vi "User Event IO.vi"() -> ()   [LabVIEW 2017]
uses:
  IMAQCV/GPIO/GPIO Pins.ctl
  <vilib>/Platform/TimedLoop/XDataNode/timing_clust.ctl
  <vilib>/Platform/TimedLoop/XDataNode/nitl_modes.ctl
  <vilib>/Platform/TimedLoop/XDataNode/wakeup.ctl
  <vilib>/platform/TimedLoop/XDataNode/XDataNode.xnode
  <vilib>/Platform/TimedLoop/XDataNode/XDNodeRunTimeDep.lvlib
  IMAQCV/PIIO.lvlib
panel:
  out "DIO4":bool
  out "DIO3":bool
  out "DIO2":bool
  out "DIO1":bool
  in  "stop":bool
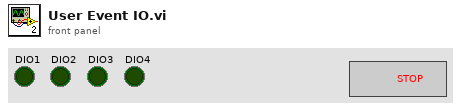
[diagram p1: front panel]
types:
  T1 = typedef "PIIO.lvlib/GPIO Pins.ctl" = u8
  T2 = cluster{"GPIO":T1[], "MODE":enum8{"INPUT", "OUTPUT"}[]}
  T3 = typedef "XDNodeRunTimeDep.lvlib/timing_clust.ctl" = cluster{"Expected End [f-1]":u64, "Actual End [f-1]":u64, "Finished Late? [f-1]":bool, "Expected End [i-1]":u64, "Actual End [i-1]":u64, "Finished Late? [i-1]":bool, "Expected Start [i]":u64, "Actual Start [i]":u64, "Expected Start [f]":u64, "Actual Start [f]":u64, "Source Name":string, "Structure Name":string, "Period":i64, "Deadline":i64, "Offset":i64, "Start":i64, "Priority":i32, "Timeout":i32, "Mode":T4, "Wakeup Reason":T5, "Error":errorcluster, "Source Type":string, "Secondary Source Type":string, "Global End Time":u64, "Global Start Time":u64, "Frame Duration":u64, "Iteration Duration":u64, "Assigned CPU":i32, "I/O Scan Engine Mode":u32}
  T4 = typedef "XDNodeRunTimeDep.lvlib/nitl_modes.ctl" = enum32{"No Change", "Process missed periods, maintain original phase", "Discard missed periods, maintain original phase", "Process missed periods, ignore original phase", "Discard missed periods, ignore original phase"}
  T5 = typedef "XDNodeRunTimeDep.lvlib/wakeup.ctl" = enum32{"Normal", "Aborted", "Asynchronous wakeup", "Timing source error", "Timed loop error", "Timeout"}
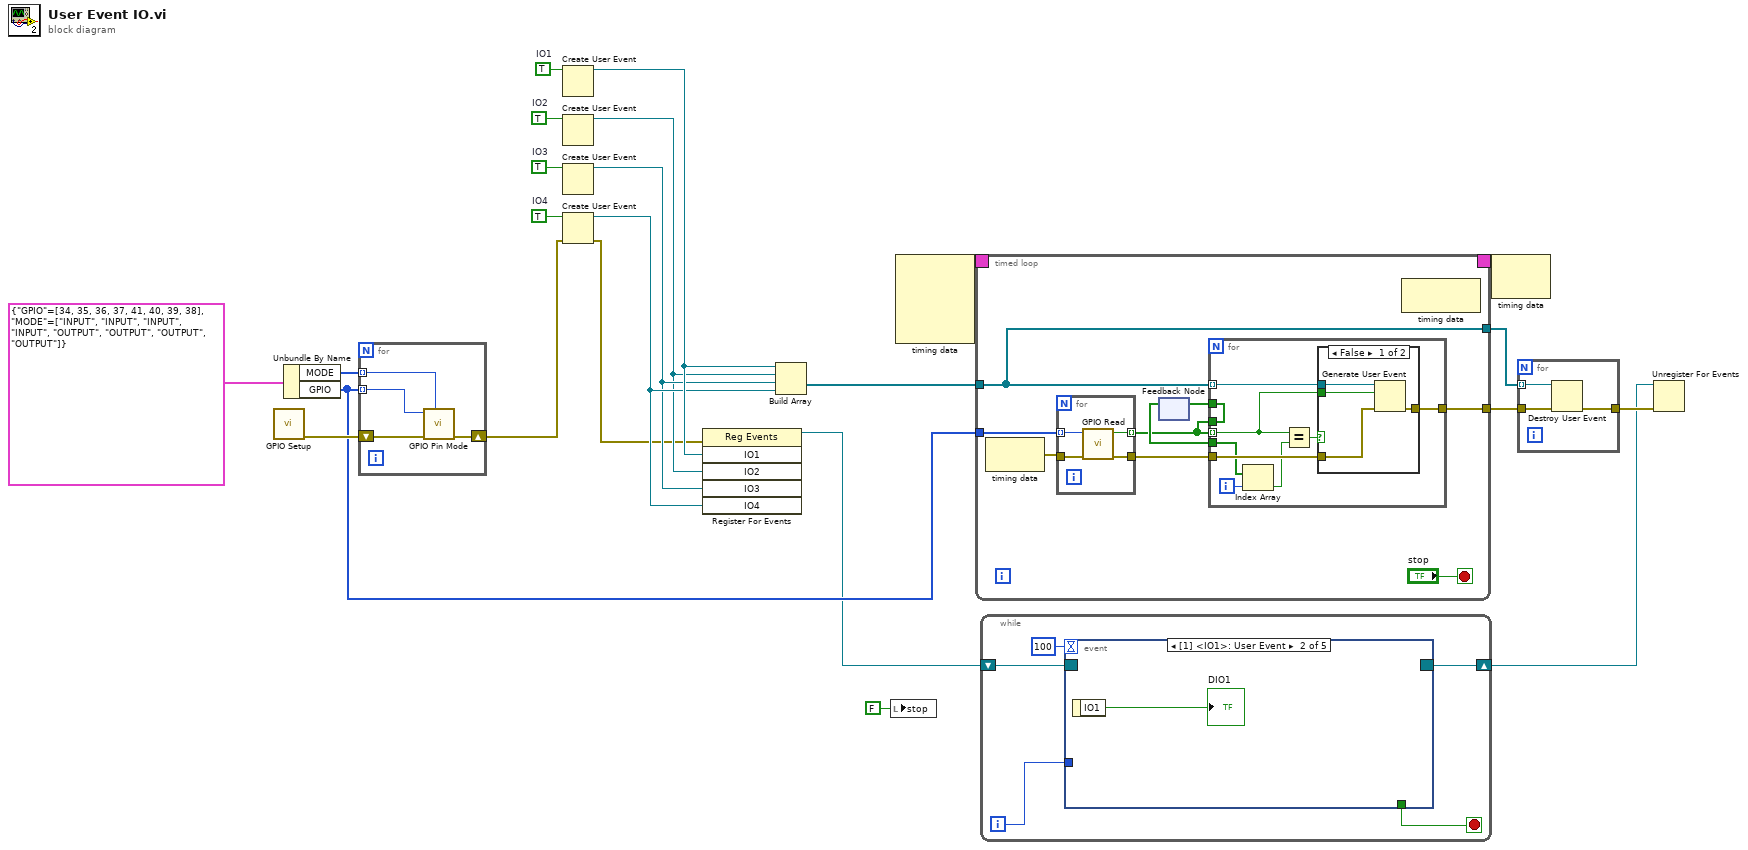
[diagram p0: block diagram]
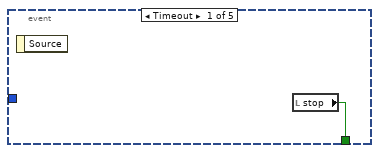
[diagram p3: hidden frame]
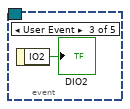
[diagram p4: hidden frame]
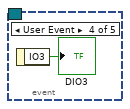
[diagram p5: hidden frame]
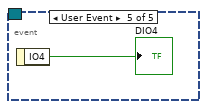
[diagram p6: hidden frame]
diagram:
  w15 = TRUE  # IO4
  w16 = TRUE  # IO3
  w17 = TRUE  # IO2
  w18 = TRUE  # IO1
  n1 = call "GPIO Setup.vi"() -> ("error out"=w19:errorcluster)  [unwired: 11 in]
  n2 = Unbundle By Name(T2 {"GPIO"=[34, 35, 36, 37, 41, 40, 39, 38], "MODE"=[enum."INPUT", enum."INPUT", enum."INPUT", enum."INPUT", enum."OUTPUT", enum."OUTPUT", enum."OUTPUT", enum."OUTPUT"]} ("GPIO")) -> ("MODE"=w3:enum8{"INPUT", "OUTPUT"}[], "GPIO"=w9:T1[])
  n3 = for {
    shift-right: [w26] -> w2
    shift-left: w19 -> [w27]
    tunnel: w9 -> [w25] mode=indexing
    tunnel: w3 -> [w24] mode=indexing
    n4 = call "GPIO Pin Mode.vi"("Pin Mode"=w24, "error in (no error)"=w27, "GPIO"=w25) -> ("error out"=w26:errorcluster)  [unwired: 8 in]
  }
  n5 = Create User Event(user event datatype=w18) -> (user event=w14:refnum<user-event>)  [unwired: 1 in, 1 out]
  n6 = Create User Event(user event datatype=w17) -> (user event=w11:refnum<user-event>)  [unwired: 1 in, 1 out]
  n7 = Create User Event(user event datatype=w16) -> (user event=w12:refnum<user-event>)  [unwired: 1 in, 1 out]
  n8 = Create User Event(user event datatype=w15, error in=w2) -> (user event=w13:refnum<user-event>, error out=w1:errorcluster)
  n9 = register-events(error in=w1, w14, w11, w12, w13) -> (reference out=w8:refnum<event-registration>)  [unwired: 1 in, 1 out]
  n10 = Build Array(w14, w11, w12, w13) -> (w10:refnum<user-event>[])
  n11 = local write "stop"(FALSE ("stop")) -> ()
  n12 = node-c288() -> (w21:T3)  [unwired: 4 in]
  n13 = timed-loop {
    tunnel: [w35] -> w22
    timing: w21 -> [_]
    timing-out: [_] -> w20
    tunnel: w10 -> [w33]
    tunnel: w9 -> [w34]
    tunnel: [w33] -> w5
    stop <- "stop" stop-if-true
    n14 = node-c288() -> (w32:errorcluster)  [unwired: 1 in]
    n15 = for {
      tunnel: w34 -> [w54] mode=indexing
      tunnel: [w52] -> w29 mode=indexing
      tunnel: w32 -> [w53]
      tunnel: [w51] -> w30
      n16 = call "GPIO Read.vi"("error in (no error)"=w53, "GPIO"=w54) -> ("error out"=w51:errorcluster, "Status"=w52:bool)  [unwired: 8 in]
    }
    n17 = feedback #1() -> (w31:bool[])  [unwired: 1 in]
    n18 = for {
      tunnel: w33 -> [w44] mode=indexing
      tunnel: w31 -> [w38]
      tunnel: w29 -> [w42] mode=indexing
      tunnel: w30 -> [w41]
      tunnel: [w45] -> w35
      tunnel: w29 -> [w40]
      tunnel: [w40] -> w28
      i -> [w39]
      n19 = Index Array(array=w38, index=w39) -> (element=w37:bool)
      n20 = Equal?(x=w42, y=w37) -> (x = y?=w43:bool)
      n21 = case shown="False" w43 {
        tunnel: w44 -> [w49 _]
        tunnel: w42 -> [w46 _]
        tunnel: w41 -> [w48 w50]
        tunnel: [w47 w50] -> w45
        frame False {
          n22 = Generate User Event(user event=w49, event data cluster=w46, error in=w48) -> (error out=w47:errorcluster)  [unwired: 1 in, 1 out]
        }
        frame True {
        }
      }
    }
    n23 = feedback-in #1(w28) -> ()
    n24 = node-c288() -> ()  [unwired: 1 in, 1 out]
  }
  n25 = while {
    shift-right: [w61] -> w6
    shift-left: w8 -> [w62]
    i -> [w58]
    stop <- w59 stop-if-true
    n26 = event shown="[1] <IO1>: User Event" {
      selector: w62 -> [_ _ _ _ _]
      dyn-events: [_ _ _ _ _] -> w61
      timeout: 100 -> [_ _ _ _ _]
      tunnel: [w63 _ _ _ _] -> w59
      tunnel: w58 -> [_ _ _ _ _]
      event Timeout {
        n27 = event-data() -> ()  [unwired: 1 in, 1 out]
        n28 = local read "stop"() -> (w63:bool)
      }
      event User Event {
        n29 = event-data() -> ("IO1"=→"DIO1":bool)  [unwired: 1 in]
      }
      event User Event {
        n30 = event-data() -> ("IO2"=→"DIO2":bool)  [unwired: 1 in]
      }
      event User Event {
        n31 = event-data() -> ("IO3"=→"DIO3":bool)  [unwired: 1 in]
      }
      event User Event {
        n32 = event-data() -> ("IO4"=→"DIO4":bool)  [unwired: 1 in]
      }
    }
  }
  n33 = node-c288(w20) -> ()  [unwired: 1 out]
  n34 = for {
    tunnel: w22 -> [w70]
    tunnel: [w69] -> w7
    tunnel: w5 -> [w68] mode=indexing
    n35 = Destroy User Event(user event=w68, error in=w70) -> (error out=w69:errorcluster)
  }
  n36 = Unregister For Events(event registration refnum=w6, error in=w7) -> ()  [unwired: 1 out]
